vi "Set Dependency.vi"(8 "error in (no error)":errorcluster, 10 "Dependency":T1, 11 "Temp01 in":refnum<class "TELLC_Temp01.lvclass">) -> (0 "error out":errorcluster, 3 "Temp01 out":refnum<class "TELLC_Temp01.lvclass">)   [LabVIEW 2017, in "TELLC_Temp01.lvclass"]
doc: "Developed by Kevin Thompson\nkevin@thompsonengineering.net\n\nCopyright 2018\nThompson Engineering, LLC"
uses:
  TELLC_Temp01.lvclass
  DataTypes/Dependency--cluster.ctl
  TELLC_Temp01.lvclass/TELLC_Temp01.ctl
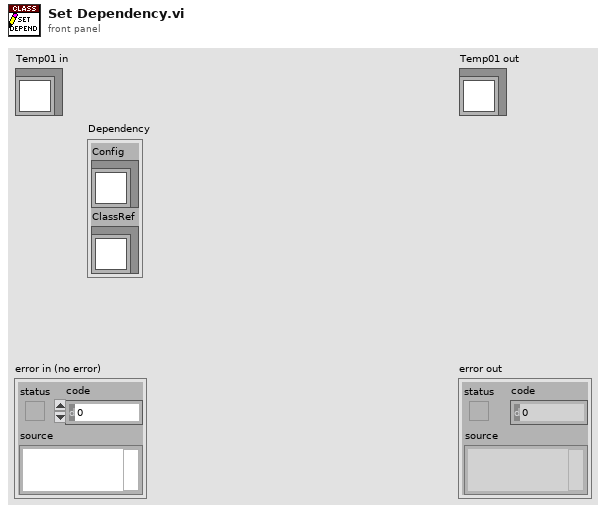
[diagram p1: front panel]
types:
  T1 = typedef "TELLC_Temp01.lvclass/Dependency--cluster.ctl" = cluster{"Config":refnum<class>, "ClassRef":refnum<class>}
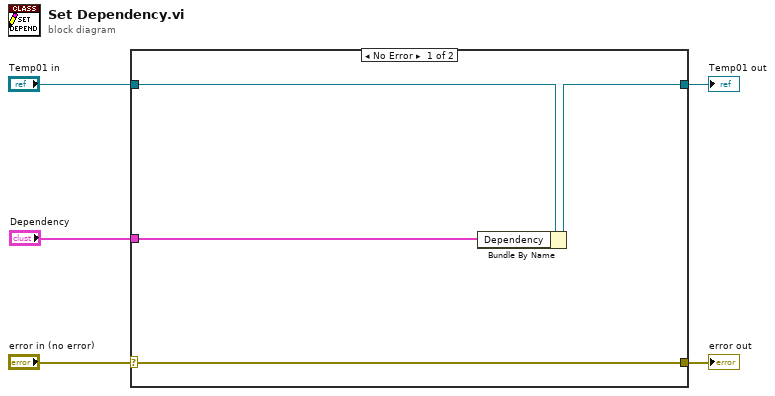
[diagram p0: block diagram]
diagram:
  n1 = case shown="No Error" "error in (no error)" {
    selector: "error in (no error)" -> [w9 w10]
    tunnel: [w9 w10] -> w4
    tunnel: [w7 w11] -> w2
    tunnel: "Temp01 in" -> [w8 w11]
    tunnel: "Dependency" -> [w6 _]
    frame No Error {
      n2 = Bundle By Name(cluster=w8, "Dependency"=w6) -> (w7:refnum<class "TELLC_Temp01.lvclass">)
    }
    frame Error {
    }
  }
  "error out" <- w4
  "Temp01 out" <- w2
